vi "DELETE_Flow Verification Calcs.vi"() -> ()   [LabVIEW 2012]
panel:
  out "Rho":string
  out "Cp":string
  out "CFM HX":string
  out "Qair":string
  out "Mdot Air":string
  out "CFM NOZZLE":string
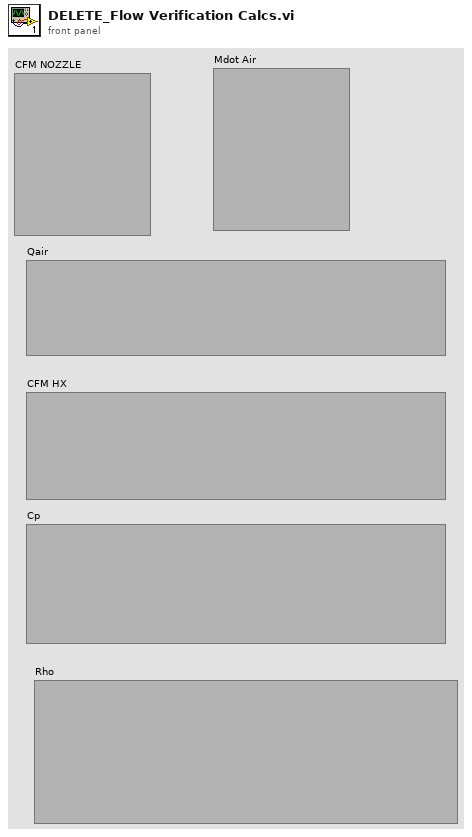
[diagram p1: front panel]
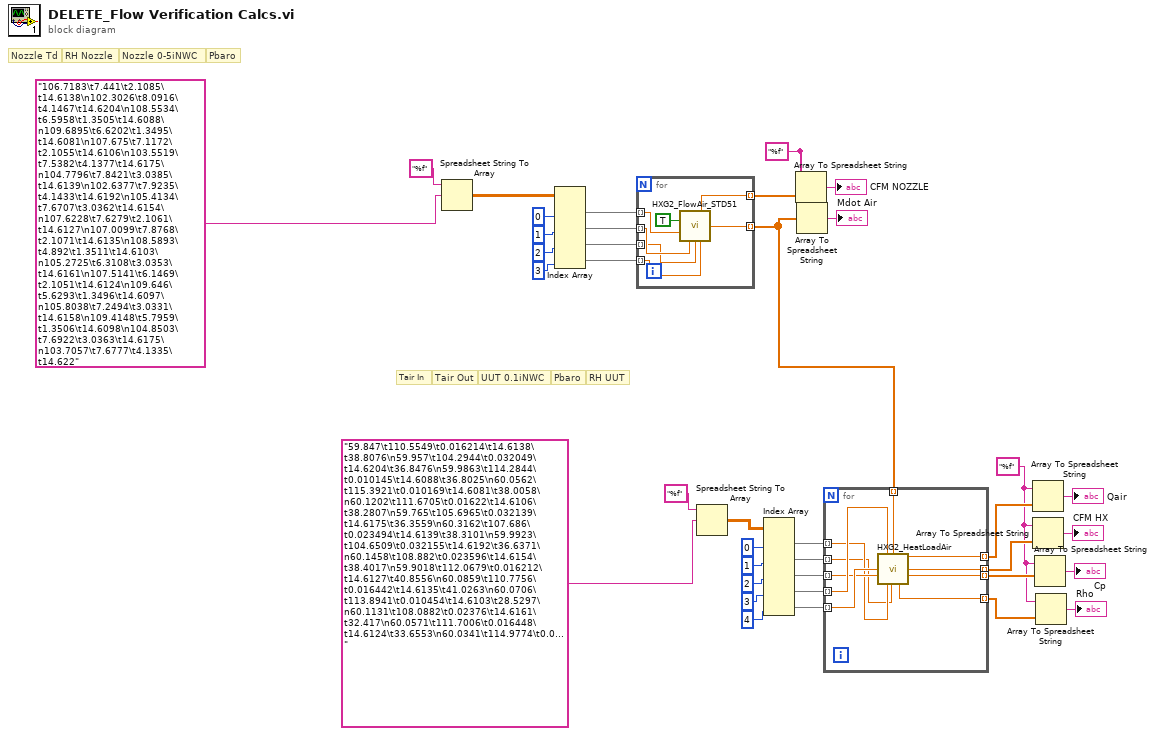
[diagram p0: block diagram]
diagram:
  w5 = "%f" ("format string")
  w25 = "%f" ("format string")
  # "Tair In"
  # "Tair Out"
  # "UUT 0.1iNWC"
  # "RH UUT"
  # "Pbaro"
  # "Pbaro"
  # "Nozzle 0-5iNWC"
  # "RH Nozzle"
  # "Nozzle Td"
  n1 = Spreadsheet String To Array(format string="%f", spreadsheet string="106.7183\t7.441\t2.1085\t14.6138\n102.3026\t8.0916\t4.1467\t14.6204\n108.5534\t6.5958\t1.3505\t14.6088\n109.6895\t6.6202\t1.3495\t14.6081\n107.675\t7.1172\t2.1055\t14.6106\n103.5519\t7.5382\t4.1377\t14.6175\n104.7796\t7.8421\t3.0385\t14.6139\n102.6377\t7.9235\t4.1433\t14.6192\n105.4134\t7.6707\t3.0362\t14.6154\n107.6228\t7.6279\t2.1061\t14.6127\n107.0099\t7.8768\t2.1071\t14.6135\n108.5893\t4.892\t1.3511\t14.6103\n105.2725\t6.3108\t3.0353\t14.6161\n107.5141\t6.1469\t2.1051\t14.6124\n109.646\t5.6293\t1.3496\t14.6097\n105.8038\t7.2494\t3.0331\t14.6158\n109.4148\t5.7959\t1.3506\t14.6098\n104.8503\t7.6922\t3.0363\t14.6175\n103.7057\t7.6777\t4.1335\t14.622") -> (array=w37:dbl[][])  [unwired: 2 in]
  n2 = Index Array(array=w37, index (col) #1=0 ("disabled index (col)"), index (col) #2=1 ("disabled index (col)"), index (col) #3=2 ("disabled index (col)"), index (col) #4=3 ("disabled index (col)")) -> (element #1=w32:dbl[], element #2=w31:dbl[], element #3=w30:dbl[], element #4=w29:dbl[])  [unwired: 4 in]
  n3 = for {
    tunnel: w32 -> [w44] mode=indexing
    tunnel: w31 -> [w43] mode=indexing
    tunnel: w30 -> [w42] mode=indexing
    tunnel: w29 -> [w41] mode=indexing
    tunnel: [w40] -> w12 mode=indexing
    tunnel: [w39] -> w28 mode=indexing
    n4 = call "HXG2_FlowAir_STD51.vi"("1.25\" Nozzle"=TRUE ("1.25\" Nozzle"), "Nozzle in Td °F"=w44, "Nozzle in %RH"=w43, "Nozzle DP inWC"=w42, "Pbarometric psi"=w41) -> ("CFM Nozzle"=w39:dbl, "Mdot (lbm/hr)"=w40:dbl)  [unwired: 5 in, 4 out]
  }
  n5 = Spreadsheet String To Array(format string="%f", spreadsheet string="59.847\t110.5549\t0.016214\t14.6138\t38.8076\n59.957\t104.2944\t0.032049\t14.6204\t36.8476\n59.9863\t114.2844\t0.010145\t14.6088\t36.8025\n60.0562\t115.3921\t0.010169\t14.6081\t38.0058\n60.1202\t111.6705\t0.01622\t14.6106\t38.2807\n59.765\t105.6965\t0.032139\t14.6175\t36.3559\n60.3162\t107.686\t0.023494\t14.6139\t38.3101\n59.9923\t104.6509\t0.032155\t14.6192\t36.6371\n60.1458\t108.882\t0.023596\t14.6154\t38.4017\n59.9018\t112.0679\t0.016212\t14.6127\t40.8556\n60.0859\t110.7756\t0.016442\t14.6135\t41.0263\n60.0706\t113.8941\t0.010454\t14.6103\t28.5297\n60.1131\t108.0882\t0.02376\t14.6161\t32.417\n60.0571\t111.7006\t0.016448\t14.6124\t33.6553\n60.0341\t114.9774\t0.010427\t14.6097\t33.0504\n60.1244\t108.6489\t0.02386\t14.6158\t37.0619\n60.0026\t114.5784\t0.010345\t14.6098\t33.7037\n60.048\t107.2058\t0.023708\t14.6175\t38.0957\n60.078\t106.0881\t0.032244\t14.622\t37.3744") -> (array=w19:dbl[][])  [unwired: 2 in]
  n6 = Index Array(array=w19, index (col) #1=0 ("disabled index (col)"), index (col) #2=1 ("disabled index (col)"), index (col) #3=2 ("disabled index (col)"), index (col) #4=3 ("disabled index (col)"), index (col) #5=4 ("disabled index (col)")) -> (element #1=w17:dbl[], element #2=w16:dbl[], element #3=w15:dbl[], element #4=w14:dbl[], element #5=w13:dbl[])  [unwired: 5 in]
  n7 = Array To Spreadsheet String(array=w28, 3:w25) -> (spreadsheet string=→"CFM NOZZLE":string)  [unwired: 1 in]
  n8 = Array To Spreadsheet String(array=w12, 3:w25) -> (spreadsheet string=→"Mdot Air":string)  [unwired: 1 in]
  n9 = for {
    tunnel: w17 -> [w51] mode=indexing
    tunnel: w16 -> [w50] mode=indexing
    tunnel: w15 -> [w52] mode=indexing
    tunnel: w14 -> [w54] mode=indexing
    tunnel: w13 -> [w53] mode=indexing
    tunnel: w12 -> [w55] mode=indexing
    tunnel: [w49] -> w7 mode=indexing
    tunnel: [w48] -> w8 mode=indexing
    tunnel: [w47] -> w6 mode=indexing
    tunnel: [w46] -> w4 mode=indexing
    n10 = call "HXG2_HeatLoadAir.vi"("Pbaro (psia)"=w54, "Mdot Air (lbm/hr)"=w55, "%RH UUT"=w53, "dP UUT (inWC)"=w52, "Air In Avg (°F)"=w51, "Air Out Avg (°F)"=w50) -> ("Q air (BTU/hr)"=w49:dbl, "CFM HX"=w48:dbl, "Moist Air Cp (BTU/lb)"=w47:dbl, "Moist Air Density (lbm/ft³)"=w46:dbl)  [unwired: 4 in, 2 out]
  }
  n11 = Array To Spreadsheet String(array=w7, 3:w5) -> (spreadsheet string=→"Qair":string)  [unwired: 1 in]
  n12 = Array To Spreadsheet String(array=w8, 3:w5) -> (spreadsheet string=→"CFM HX":string)  [unwired: 1 in]
  n13 = Array To Spreadsheet String(array=w6, 3:w5) -> (spreadsheet string=→"Cp":string)  [unwired: 1 in]
  n14 = Array To Spreadsheet String(array=w4, 3:w5) -> (spreadsheet string=→"Rho":string)  [unwired: 1 in]
